vi "Read Transfer Buffer.vi"(8 "error in (no error)":errorcluster, 10 "Transfer":refnum<class "Transfer.lvclass">, 11 "UDP Transceiver in":refnum<class "UDP Transceiver.lvclass">) -> (0 "error out":errorcluster, 1 "transfer data":string, 3 "UDP Transceiver out":refnum<class "UDP Transceiver.lvclass">)   [LabVIEW 2017, in "UDP.lvlib" / "UDP Transceiver.lvclass"]
uses:
  UDP Transceiver.lvclass
  Builds/Data Sharing Framework/Current/Core/DSF Core.lvlibp/Classes/Transfer/Transfer.lvclass
  Builds/Data Sharing Framework/Current/Core/DSF Core.lvlibp/Classes/Buffer/Read Buffer 1D U8.vi
  Builds/Data Sharing Framework/Current/Core/DSF Core.lvlibp/Classes/Buffer/Buffer.lvclass
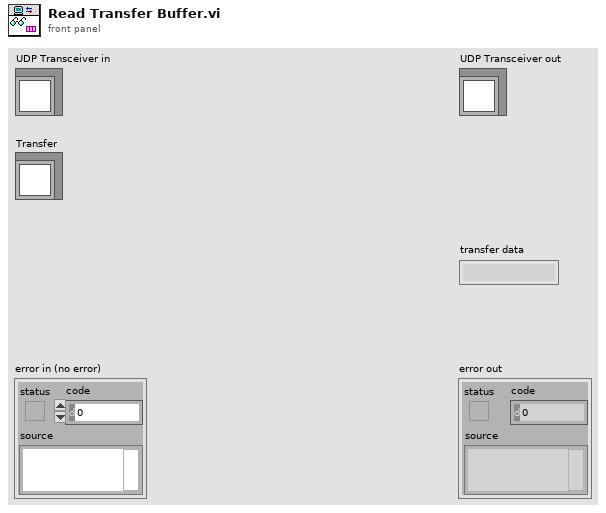
[diagram p1: front panel]
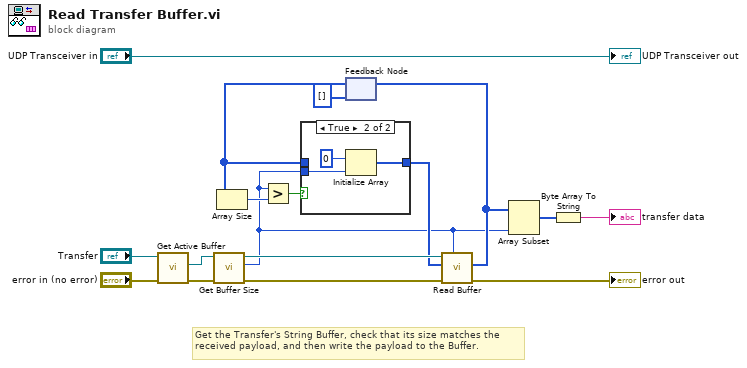
[diagram p0: block diagram]
diagram:
  # "Get the Transfer's String Buffer, check that its size matches the received payload, and then write the payload to the Buffer."
  n1 = call "Get Active Buffer.vi"("error in (no error)"="error in (no error)", "Transfer in"="Transfer") -> ("error out"=w10:errorcluster, "Buffer"=w9:refnum<class "Buffer.lvclass">)  [unwired: 7 in, 1 out]
  n2 = call "Get Buffer Size.vi"("Buffer in"=w9) -> ("buffer size"=w4:u64, "Buffer out"=w8:refnum<class "Buffer.lvclass">)  [unwired: 9 in]
  n3 = feedback #1(u8[] []) -> (w7:u8[])
  n4 = Array Size(array=w7) -> (size(s)=w12:i32)
  n5 = Greater?(x=w4, y=w12) -> (0:w11:bool)
  n6 = case shown="True" w11 {
    tunnel: w7 -> [w17 _]
    tunnel: [w17 w20] -> w6
    tunnel: w4 -> [_ w18]
    frame False {
    }
    frame True {
      n7 = Initialize Array(u8 0 ("Numeric"), w18) -> (w20:u8[])
    }
  }
  n8 = call-poly "Read Buffer.vi"("count (-1: rest)"=w4, "error in (no error)"=w10, "dst array in"=w6, "Buffer in"=w8) -> ("error out"=→"error out":errorcluster, "dst array out"=w5:u8[])  [unwired: 4 in, 2 out]
  n9 = feedback-in #1(w5) -> ()
  n10 = Array Subset(array=w5, length=w4) -> (w14:u8[])  [unwired: 1 in]
  n11 = Byte Array To String(unsigned byte array=w14) -> (string=→"transfer data":string)
  "UDP Transceiver out" <- "UDP Transceiver in"
